vi "FTPBeadScan.vi"() -> ()   [LabVIEW 2016]
uses:
  <vilib>/FTP/NI_FTP.lvlib
panel:
  in  "stop":bool
  out "error out":errorcluster
  out "file error":errorcluster
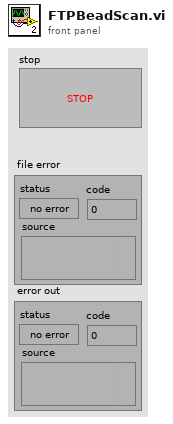
[diagram p1: front panel]
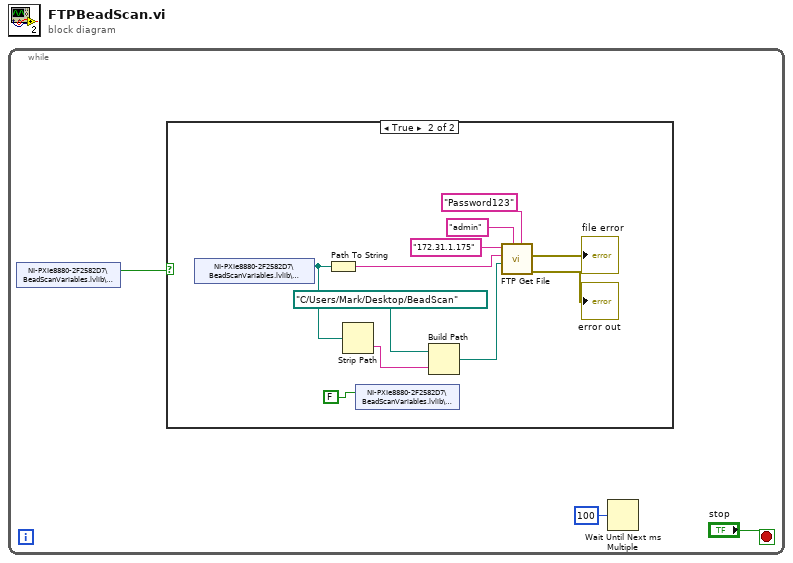
[diagram p0: block diagram]
diagram:
  n1 = while {
    stop <- "stop" stop-if-true
    n2 = shared-variable "NI-PXIe8880-2F2582D7\\BeadScanVariables.lvlib\\FileWaiting"() -> (w1:bool)  [unwired: 1 in, 1 out]
    n3 = case shown="True" w1 {
      frame False {
      }
      frame True {
        n4 = shared-variable "NI-PXIe8880-2F2582D7\\BeadScanVariables.lvlib\\BeadScanPath"() -> (w6:path)  [unwired: 1 in, 1 out]
        n5 = Path To String(path=w6) -> (string=w5:string)
        n6 = Strip Path(path=w6) -> (name=w9:string)  [unwired: 1 out]
        n7 = shared-variable "NI-PXIe8880-2F2582D7\\BeadScanVariables.lvlib\\FileWaiting"(FALSE) -> ()  [unwired: 1 in, 1 out]
        n8 = Build Path(base path=path "C:/Users/Mark/Desktop/BeadScan" ("local path"), name or relative path=w9) -> (appended path=w7:path)
        n9 = call <vilib>:"FTP Get File.vi"("password"="Password123", "user"="admin", "local path"=w7, "remote path"=w5, "host"="172.31.1.175") -> ("error out"=→"error out":errorcluster, "file error"=→"file error":errorcluster)  [unwired: 5 in]
      }
    }
    n10 = Wait Until Next ms Multiple(millisecond multiple=u32 100) -> ()  [unwired: 1 out]
  }
